vi "test Search Sub-Sections.vi"(11 "Test Case In":refnum<class "test EDS.lvclass">) -> (0 "error out":errorcluster, 3 "Test Case Out":refnum<class "test EDS.lvclass">)   [LabVIEW 2024, in "test EDS.lvclass"]
uses:
  test EDS.lvclass
  Core/EDS/EDS.lvclass
  Core/EDS/EDS.lvclass/EDS.ctl
  Core/OD Section/Section.lvclass/Section.ctl
  <vilib>/Astemes/LUnit/Test Case.lvclass/Test Case.ctl
  2a20feae-586c-4e07-ad2a-4c5ba82c9b88.vi
  <vilib>/Astemes/LUnit/Append Pass Result.vi
  <vilib>/Astemes/LUnit/Append Fail Result.vi
  <vilib>/Astemes/LUnit/Describe Comparison.vi
  2a20feae-586c-4e07-ad2a-4c5ba82c9b88.vi/9c5d11cd-9439-4240-a1ee-d9baace9c924.vi
  <vilib>/Astemes/LUnit/Run In UI.vi
  <vilib>/Utility/error.llb/Clear Errors.vi
  <vilib>/Astemes/LUnit/Describe Variant.vi
  test EDS.lvclass/test EDS.ctl
  Core/Object Dictionary/Dictionary.lvclass
  Core/OD Section/Section.lvclass
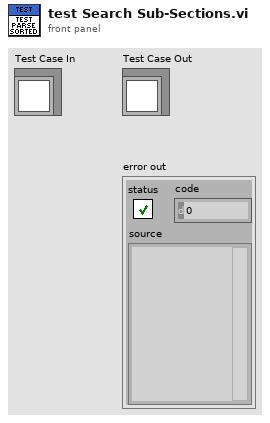
[diagram p1: front panel]
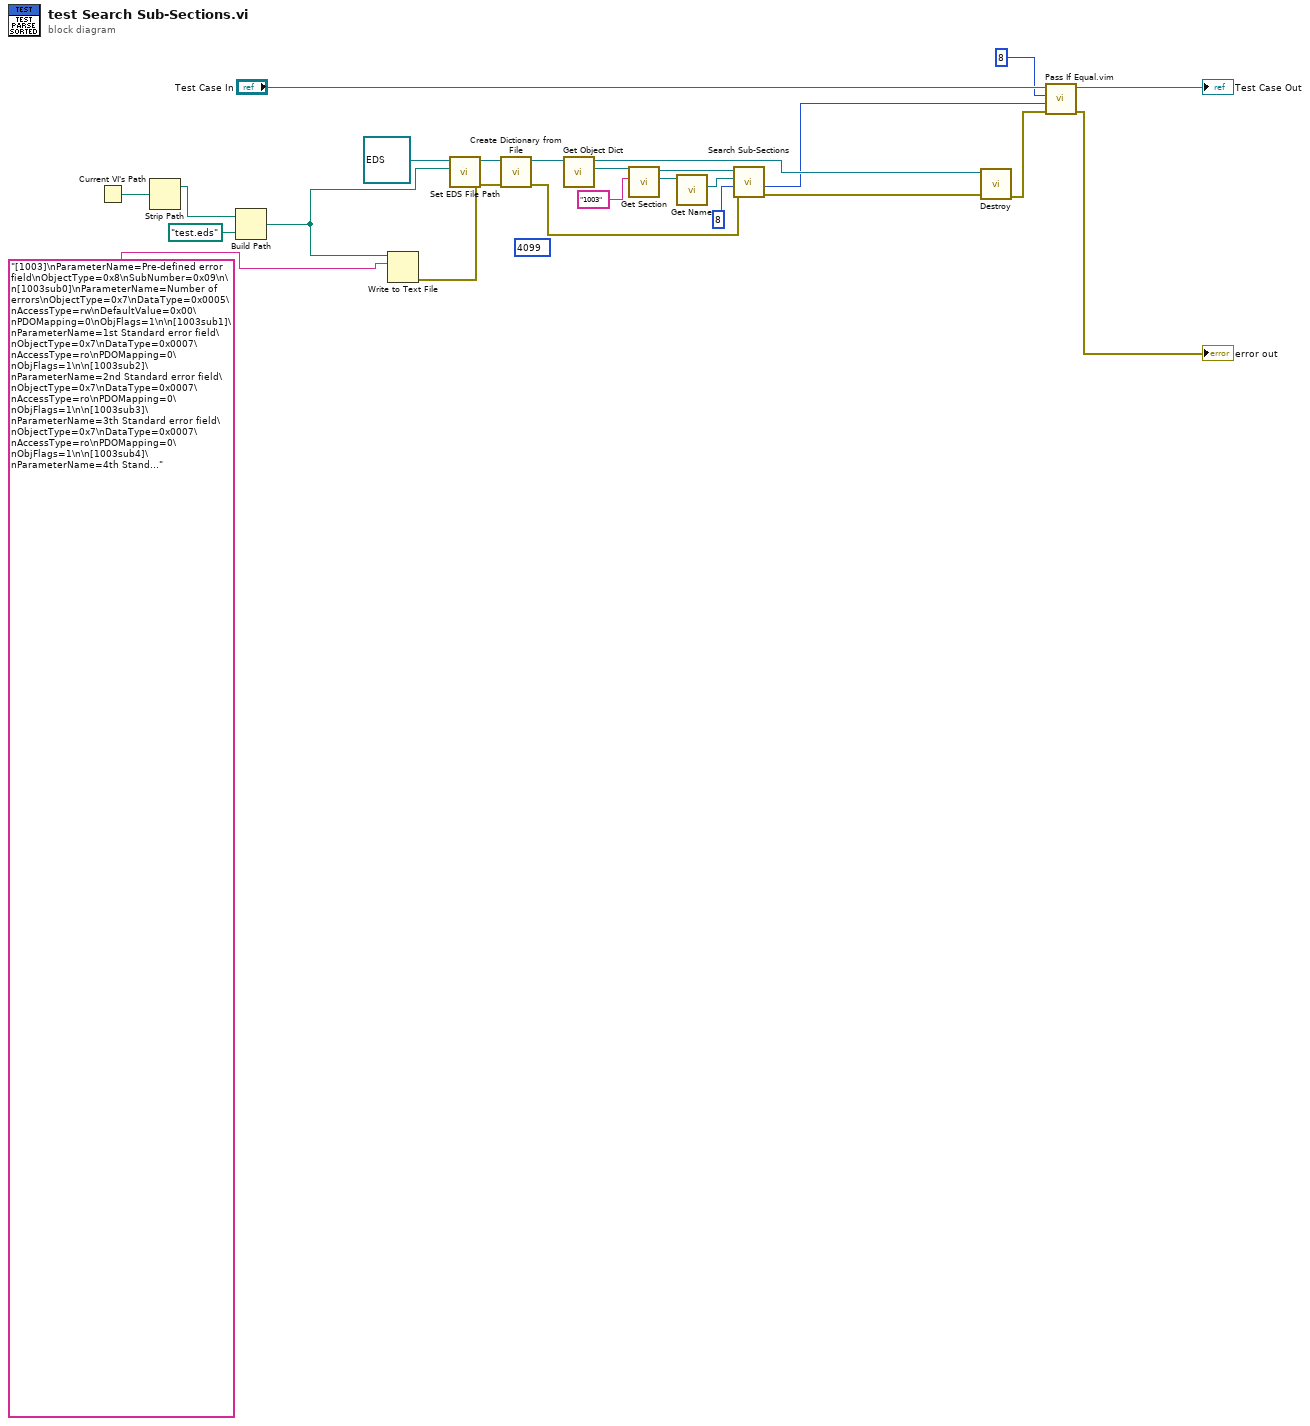
[diagram p0: block diagram]
diagram:
  (unwired) u16 4099 ("Numeric")
  n1 = Current VI's Path() -> (path=w19:path)
  n2 = Strip Path(path=w19) -> (stripped path=w15:path)  [unwired: 1 out]
  n3 = Build Path(base path=w15, name or relative path=path "test.eds") -> (appended path=w16:path)
  n4 = Write to Text File(file (use dialog)=w16, text="[1003]\nParameterName=Pre-defined error field\nObjectType=0x8\nSubNumber=0x09\n\n[1003sub0]\nParameterName=Number of errors\nObjectType=0x7\nDataType=0x0005\nAccessType=rw\nDefaultValue=0x00\nPDOMapping=0\nObjFlags=1\n\n[1003sub1]\nParameterName=1st Standard error field\nObjectType=0x7\nDataType=0x0007\nAccessType=ro\nPDOMapping=0\nObjFlags=1\n\n[1003sub2]\nParameterName=2nd Standard error field\nObjectType=0x7\nDataType=0x0007\nAccessType=ro\nPDOMapping=0\nObjFlags=1\n\n[1003sub3]\nParameterName=3th Standard error field\nObjectType=0x7\nDataType=0x0007\nAccessType=ro\nPDOMapping=0\nObjFlags=1\n\n[1003sub4]\nParameterName=4th Standard error field\nObjectType=0x7\nDataType=0x0007\nAccessType=ro\nPDOMapping=0\nObjFlags=1\n\n[1003sub5]\nParameterName=5th Standard error field\nObjectType=0x7\nDataType=0x0007\nAccessType=ro\nPDOMapping=0\nObjFlags=1\n\n[1003sub6]\nParameterName=6th Standard error field\nObjectType=0x7\nDataType=0x0007\nAccessType=ro\nPDOMapping=0\nObjFlags=1\n\n[1003sub7]\nParameterName=7th Standard error field\nObjectType=0x7\nDataType=0x0007\nAccessType=ro\nPDOMapping=0\nObjFlags=1\n\n[1003sub8]\nParameterName=8th Standard error field\nObjectType=0x7\nDataType=0x0007\nAccessType=ro\nPDOMapping=0\nObjFlags=1") -> (error out=w17:errorcluster)  [unwired: 2 in, 2 out]
  n5 = call "Set EDS File Path.vi"("EDS File Path"=w16, "EDS in"=refnum<class "EDS.lvclass"> refnum ("EDS.lvlib:EDS.lvclass")) -> ("EDS out"=w20:refnum<class "EDS.lvclass">)  [unwired: 9 in]
  n6 = call "Create Dictionary from File.vi"("error in"=w17, "EDS in"=w20) -> ("error out"=w5:errorcluster, "EDS out"=w12:refnum<class "EDS.lvclass">)  [unwired: 8 in]
  n7 = call "Get Object Dict.vi"("EDS in"=w12) -> ("Object Dictionary"=w11:refnum<class "Dictionary.lvclass">, "EDS out"=w3:refnum<class "EDS.lvclass">)  [unwired: 9 in]
  n8 = call "Get Section.vi"("Section"="1003", "Dictionary in"=w11) -> ("Section out"=w8:refnum<class "Section.lvclass">, "Dictionary out"=w10:refnum<class "Dictionary.lvclass">)  [unwired: 7 in, 1 out]
  n9 = call "Get Name.vi"("Object Entry in"=w8) -> ("Section Name"=w7:refnum<class "Section Name.lvclass">)  [unwired: 9 in, 1 out]
  n10 = call "Search Sub-Sections.vi"("error in"=w5, "Count"=u8 8, "Parent Section"=w7, "Dictionary in"=w10) -> ("error out"=w4:errorcluster, "Found"=w1:u8)  [unwired: 4 in, 2 out]
  n11 = call "Destroy.vi"("error in"=w4, "EDS in"=w3) -> ("error out"=w13:errorcluster)  [unwired: 8 in, 1 out]
  n12 = call "Pass If Equal.vim"("error in (no error)"=w13, "Actual"=w1, "Expected"=u8 8 ("Count"), "LUnit Test Case In"="Test Case In") -> ("error out"=→"error out":errorcluster, "LUnit Test Case Out"=→"Test Case Out":refnum<class "test EDS.lvclass">)  [unwired: 6 in]
